vi "SendUDPEth.vi"(0 "connection ID":refnum<k16>, 1 "Msg":T1, 2 "Port":u16, 4 "IP":string="127.0.0.1") -> (6 "status":bool)   [LabVIEW 2017]
panel:
  out "error out":errorcluster
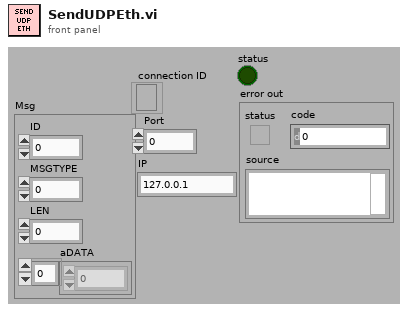
[diagram p1: front panel]
types:
  T1 = cluster{"ID":u32, "MSGTYPE":u8, "LEN":u8, "aDATA":u8[]}
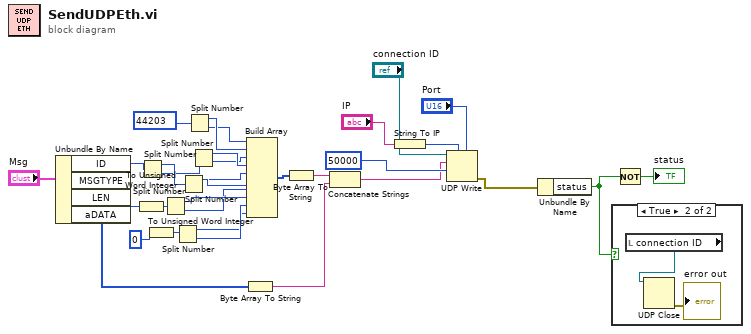
[diagram p0: block diagram]
diagram:
  n1 = Unbundle By Name("Msg") -> ("ID"=w13:u32, "LEN"=w18:u8, "aDATA"=w31:u8[])  [unwired: 1 out]
  n2 = To Unsigned Word Integer(number=w18) -> (unsigned 16bit integer=w17:u16)
  n3 = Split Number(x=w13) -> (hi(x)=w24:u16, lo(x)=w19:u16)
  n4 = To Unsigned Word Integer(number=u32 0 ("x")) -> (unsigned 16bit integer=w8:u16)
  n5 = Split Number(x=w17) -> (hi(x)=w16:u8, lo(x)=w12:u8)
  n6 = Split Number(x=w8) -> (hi(x)=w10:u8, lo(x)=w11:u8)
  n7 = Split Number(x=w24) -> (hi(x)=w21:u8, lo(x)=w20:u8)
  n8 = Split Number(x=u16 44203 ("element")) -> (hi(x)=w27:u8, lo(x)=w26:u8)
  n9 = Split Number(x=w19) -> (hi(x)=w23:u8, lo(x)=w22:u8)
  n10 = Byte Array To String(unsigned byte array=w31) -> (string=w28:string)
  n11 = Build Array(w26, w27, w22, w23, w20, w21, w12, w16, w11, w10) -> (w30:u8[])
  n12 = Byte Array To String(unsigned byte array=w30) -> (string=w29:string)
  n13 = Concatenate Strings(w29, w28) -> (w3:string)
  n14 = String To IP(1:"IP") -> (0:w1:u32)
  n15 = UDP Write(address=w1, port or service name="Port", connection ID="connection ID", data in=w3, 9:50000 ("timeout ms (25000)")) -> (error out=w4:errorcluster)  [unwired: 1 in, 1 out]
  n16 = Unbundle By Name(w4) -> ("status"=w15:bool)
  n17 = case shown="True" w15 {
    frame False {
    }
    frame True {
      n18 = local read "connection ID"() -> (w34:refnum<k16>)
      n19 = UDP Close(connection ID=w34) -> (error out=→"error out":errorcluster)  [unwired: 1 in, 1 out]
    }
  }
  n20 = Not(x=w15) -> (.not. x?=→"status":bool)
